vi "SeparateHeaderAndData.vi"(3 "File Text":string) -> (0 "data":dbl[][](array[numeric]), 1 "Header Text":string[](array[string]))   [LabVIEW 2014]
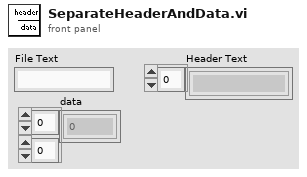
[diagram p1: front panel]
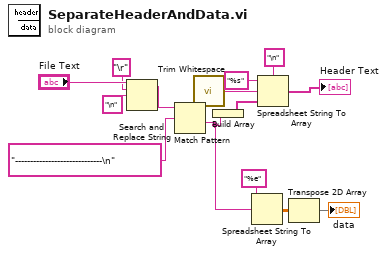
[diagram p0: block diagram]
diagram:
  n1 = Search and Replace String(input string="File Text", search string="\r", replace string="\n") -> (result string=w10:string)  [unwired: 5 in, 3 out]
  n2 = Match Pattern(string=w10, regular expression="-----------------------------\n" ("format string")) -> (before substring=w6:string, after substring=w2:string)  [unwired: 1 in, 2 out]
  n3 = call <vilib>:"Trim Whitespace.vi"("string"=w6) -> ("trimmed string"=w14:string)  [unwired: 1 in]
  n4 = Build Array(w2) -> (w7:string[])
  n5 = Spreadsheet String To Array(format string="%e", spreadsheet string=w2) -> (array=w3:dbl[][])  [unwired: 2 in]
  n6 = Spreadsheet String To Array(delimiter (Tab)="\n", format string="%s", spreadsheet string=w14, array type (2D Dbl)=w7) -> (array=→"Header Text":string[])
  n7 = Transpose 2D Array(2D array=w3) -> (transposed array=→"data":dbl[][])
